vi "禹山pH_获取温度和测量值.vi"(8 "error in (no error)":errorcluster caption="错误输入（无错误）", 11 "MB session in":refnum<class "MB_Master.lvclass">) -> (0 "error out":errorcluster caption="错误输出", 2 "输出值":cluster{"温度测量值":sgl, "ORP":sgl, "pH":sgl}, 3 "MB session out":refnum<class "MB_Master.lvclass">)   [LabVIEW 2016, in "斯坦道多参数.lvlib"]
uses:
  <vilib>/Plasmionique/MB Master/MB_Master/MB_Master.lvclass
  <vilib>/Plasmionique/MB Master/MB Master.lvlib
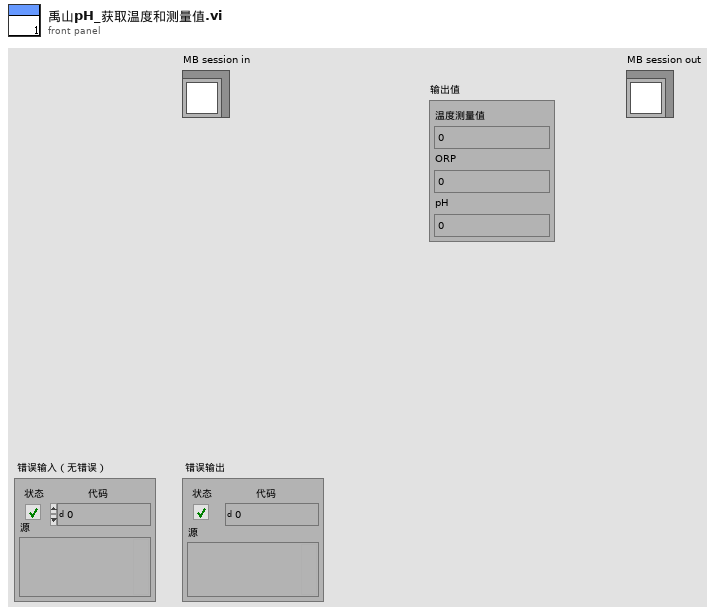
[diagram p1: front panel]
types:
  T1 = cluster{"pH":u32, "DO":u32, "Cond":u32, "Turb":u32, "叶绿素a":u32, "藻密度":u32, "ORP":u32}
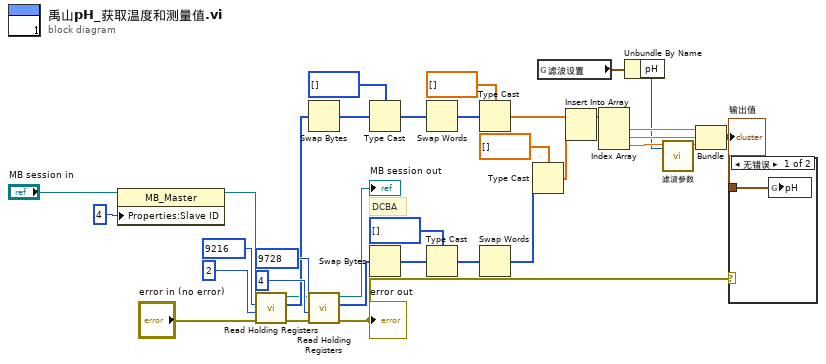
[diagram p0: block diagram]
diagram:
  # "DCBA"
  n1 = property class="MB_Master"(reference="MB session in", "Properties:Slave ID"=u16 4 ("y")) -> (reference out=w11:refnum<class "MB_Master.lvclass">)  [unwired: 1 in, 1 out]
  n2 = call <vilib>:"Read Holding Registers.vi"("error in (no error)"="error in (no error)", "quantity"=u16 2, "starting address"=u16 9216, "MB session in"=w11) -> ("error out"=w12:errorcluster, "Registers"=w15:u16[], "MB session out"=w10:refnum<class "MB_Master.lvclass">)  [unwired: 5 in]
  n3 = Swap Bytes(anything=w15) -> (byte swapped=w20:u16[])
  n4 = call <vilib>:"Read Holding Registers.vi"("error in (no error)"=w12, "quantity"=u16 4, "starting address"=u16 9728, "MB session in"=w10) -> ("error out"=w14:errorcluster, "Registers"=w27:u16[], "MB session out"=→"MB session out":refnum<class "MB_Master.lvclass">)  [unwired: 5 in]
  "error out" <- w14
  n5 = Type Cast(type=u32[] [] ("数组 2"), x=w20) -> (*(type *) &x=w18:u32[])
  n6 = Swap Bytes(anything=w27) -> (byte swapped=w26:u16[])
  n7 = Swap Words(1:w18) -> (0:w16:u32[])
  n8 = Type Cast(type=u32[] [] ("数组 2"), x=w26) -> (*(type *) &x=w30:u32[])
  n9 = Type Cast(type=sgl[] [] ("数组 2"), x=w16) -> (*(type *) &x=w9:sgl[])
  n10 = Swap Words(1:w30) -> (0:w32:u32[])
  n11 = Type Cast(type=sgl[] [] ("数组 2"), x=w32) -> (*(type *) &x=w7:sgl[])
  n12 = global read "断电保存变量.vi" "滤波设置"() -> (w2:T1)
  n13 = Insert Into Array(array=w9, new element=w7) -> (w8:sgl[])  [unwired: 1 in]
  n14 = Index Array(array=w8) -> (element #1=w25:sgl, element #2=w24:sgl, element #3=w4:sgl)  [unwired: 3 in]
  n15 = Unbundle By Name(w2) -> ("pH"=w1:u32)
  n16 = call "滤波参数.vi"("滤波次数"=w1, "x"=w4) -> ("mode"=w3:dbl)  [unwired: 9 in]
  n17 = Bundle("数值"=w25, "数值"=w24, "mode"=w3) -> (w23:cluster{"数值":sgl, "数值":sgl, "mode":dbl})  [unwired: 1 in]
  "输出值" <- w23
  n18 = case shown="无错误" w14 {
    tunnel: w23 -> [w35 _]
    frame No Error {
      n19 = global write "禹山过程全局变量.vi" "pH"(w35) -> ()
    }
    frame Error {
    }
  }
